vi "Data_Convert.vi"(1 "string":string, 2 "ID":string) -> (0 "CAN frame":T1 {"payload" format="%x"; "timestamp" format="%<%.7X\n%x>T"; "type" items=["CAN Data"=0, "CAN Remote"=1, "CAN Bus Error"=2, "CAN 2.0 Data"=8, "CAN FD Data"=16, "CAN FD+BRS Data"=24, "J1939 Data"=192, "Delay"=224, "Log Trigger"=225, "Start Trigger"=226]; "identifier" format="%x"})   [LabVIEW 2023]
uses:
  <vilib>/xnet/xnet.llb/XNET Frame CAN.ctl
  <vilib>/xnet/xnet.llb/XNET Frame Type CAN.ctl
  C:/Elatch-Bench-Test/VIs 64 bits/Users/k90011005/Desktop/Practicas/C#/String-Hexa/bin/Debug/String-Hexa.dll
  VIs 64 bits/Users/k90011005/Desktop/Practicas/C#/String-Hexa/bin/Debug/String-Hexa.dll
panel:
  out "unsigned byte array":u8[](array[numeric]) format="%x"
  out "number":u32 format="%x"
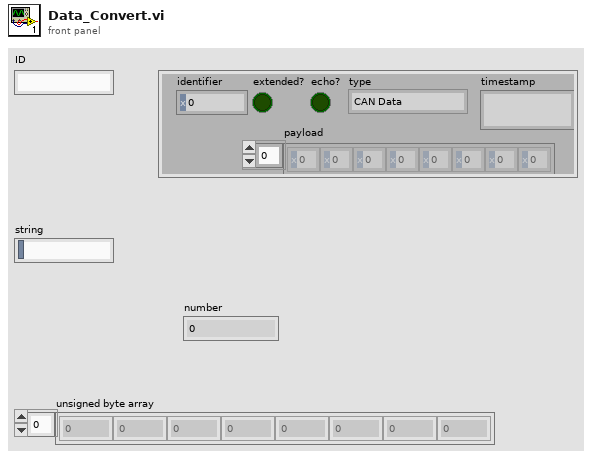
[diagram p1: front panel]
types:
  T1 = typedef "XNET Frame CAN.ctl" = cluster{"timestamp":timestamp, "payload":u8[], "identifier":u32, "type":T2, "extended?":bool, "echo?":bool}
  T2 = typedef "XNET Frame Type CAN.ctl" = u8
  T3 = cluster{"timestamp":timestamp, "StringToByteArray":u8[], u32, "type":T2, "Extended":bool, "Echo":bool}
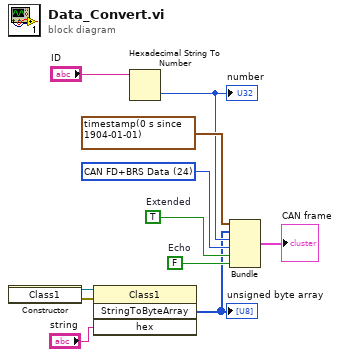
[diagram p0: block diagram]
diagram:
  w8 = T2 24 items=["CAN Data"=0, "CAN Remote"=1, "CAN Bus Error"=2, "CAN 2.0 Data"=8, "CAN FD Data"=16, "CAN FD+BRS Data"=24, "J1939 Data"=192, "Delay"=224, "Log Trigger"=225, "Start Trigger"=226] ("type")
  w6 = FALSE  # Echo
  w7 = TRUE  # Extended
  n1 = constructor class="Class1"() -> (reference out=w4:refnum<k24>, error out=w3:errorcluster)  [unwired: 3 in, 1 out]
  n2 = invoke class="Class1" method="StringToByteArray"(reference=w4, error in=w3, "hex"="string") -> ("StringToByteArray"=w1:u8[])  [unwired: 1 in, 3 out]
  "unsigned byte array" <- w1
  n3 = Hexadecimal String To Number(string="ID") -> (number=w9:u32)  [unwired: 2 in, 1 out]
  "number" <- w9
  n4 = Bundle("timestamp"=timestamp(0 s since 1904-01-01), "StringToByteArray"=w1, w9, "type"=w8, "Extended"=w7, "Echo"=w6) -> (→"CAN frame":T3)  [unwired: 1 in]
